vi "dvp Vi Get Bayer Decode Sel.vi"(10 "pBayerDecodeSel":u32, 11 "handle":u32) -> (2 "pBayerDecodeSel out":u32, 3 "function return":u32(ring))   [LabVIEW 2018, in "LabViewDVPCamera.lvlib"]
doc: "LabviewDvp2Api dvpStatus dvpViGetBayerDecodeSel(dvpHandle handle, dvpUint32 *pBayerDecodeSel);"
uses:
  LabViewDVPCamera.lvlib
  LabViewDVPCamera/LabViewDVPCamera.dll
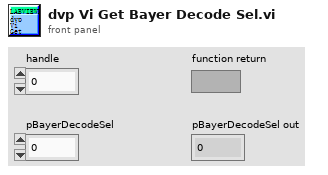
[diagram p1: front panel]
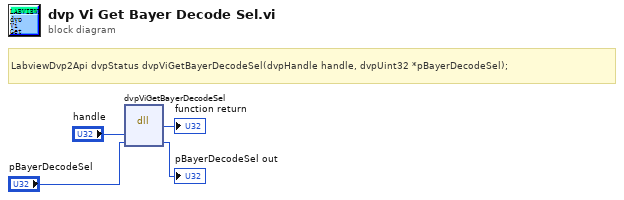
[diagram p0: block diagram]
diagram:
  # "LabviewDvp2Api dvpStatus dvpViGetBayerDecodeSel(dvpHandle handle, dvpUint32 *pBayerDecodeSel);"
  n1 = dll-call lib="C:/Program Files (x86)/DVP2 Labview cn 64/Sample/LabViewDVPCamera/LabViewDVPCamera.*" fn="dvpViGetBayerDecodeSel"("handle"="handle", "pBayerDecodeSel"="pBayerDecodeSel") -> (→"function return":u32, "pBayerDecodeSel"=→"pBayerDecodeSel out":u32)  [unwired: 4 in, 2 out]
